vi "WBRT Convert SPI Data.vi"(11 "Read Data":u8[](array[numeric])) -> (3 "Value":i16)   [LabVIEW 2012]
doc: "Converts SPI data in the form of 2 U8s to a sing I16 value. This data is later scaled and reported as either gyro or acceleration data.\n\nAuthor: Brandon Steele\n\nCopyright: Brigham Young University"
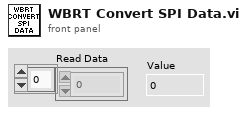
[diagram p1: front panel]
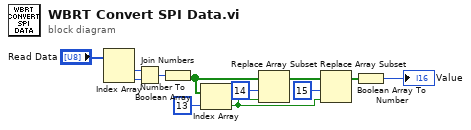
[diagram p0: block diagram]
diagram:
  n1 = Index Array(array="Read Data") -> (element #1=w3:u8, element #2=w2:u8)  [unwired: 2 in]
  n2 = Join Numbers(hi=w3, lo=w2) -> ((hi.lo)=w5:u16)
  n3 = Number To Boolean Array(number=w5) -> (Boolean array=w11:bool[])
  n4 = Index Array(array=w11, index=13) -> (element=w7:bool)
  n5 = Replace Array Subset(array=w11, new element=w7, index=14) -> (w8:bool[])
  n6 = Replace Array Subset(array=w8, new element=w7, index=15) -> (w6:bool[])
  n7 = Boolean Array To Number(Boolean array=w6) -> (number=→"Value":i16)
